vi "Excel Report - Graph Generation.vi"() -> ()   [LabVIEW 2023]
doc: "This example shows how to insert a bar graph into an Excel workbook and to set the value number format to \"percent\"."
uses:
  <vilib>/Utility/NIReport.llb/Report Type.ctl
  <vilib>/Utility/NIReport.llb/NI_report.lvclass
  <vilib>/Utility/NIReport.llb/Excel/NI_Excel.lvclass
  <vilib>/Utility/NIReport.llb/NI_ReportGenerationCore.lvlib
panel:
  in  "Has Legend?":bool
  in  "Graph Type":i32(ring)=51 items=["xlColumnClustered"=51, "xlColumnStacked"=52, "xlColumnStacked100"=53, "xl3DColumnClustered"=54, "xl3DColumnStacked"=55, "xl3DColumnStacked100"=56, "xlBarClustered"=57, "xlBarStacked"=58, "xlBarStacked100"=59, "xl3DBarClustered"=60, "xl3DBarStacked"=61, "xl3DBarStacked100"=62, "xlLineStacked"=63, "xlLineStacked100"=64, "xlLineMarkers"=65, "xlLineMarkersStacked"=66, "xlLineMarkersStacked100"=67, "xlPieOfPie"=68, "xlPieExploded"=69, "xl3DPieExploded"=70, "xlBarOfPie"=71, "xlXYScatterSmooth"=72, "xlXYScatterSmoothNoMarkers"=73, "xlXYScatterLines"=74, "xlXYScatterLinesNoMarkers"=75, "xlAreaStacked"=76, "xlAreaStacked100"=77, "xl3DAreaStacked"=78, "xl3DAreaStacked100"=79, "xlDoughnutExploded"=80, "xlRadarMarkers"=81, "xlRadarFilled"=82, "xlSurface"=83, "xlSurfaceWireframe"=84, "xlSurfaceTopView"=85, "xlSurfaceTopViewWireframe"=86, "xlBubble"=15, "xlBubble3DEffect"=87, "xlStockHLC"=88, "xlStockOHLC"=89, "xlStockVHLC"=90, "xlStockVOHLC"=91, "xlCylinderColClustered"=92, "xlCylinderColStacked"=93, "xlCylinderColStacked100"=94, "xlCylinderBarClustered"=95, "xlCylinderBarStacked"=96, "xlCylinderBarStacked100"=97, "xlCylinderCol"=98, "xlConeColClustered"=99, "xlConeColStacked"=100, "xlConeColStacked100"=101, "xlConeBarClustered"=102, "xlConeBarStacked"=103, "xlConeBarStacked100"=104, "xlConeCol"=105, "xlPyramidColClustered"=106, "xlPyramidColStacked"=107, "xlPyramidColStacked100"=108, "xlPyramidBarClustered"=109, "xlPyramidBarStacked"=110, "xlPyramidBarStacked100"=111, "xlPyramidCol"=112, "xl3DColumn"=-4100, "xlLine"=4, "xl3DLine"=-4101, "xl3DPie"=-4102, "xlPie"=5, "xlXYScatter"=-4169, "xl3DArea"=-4098, "xlArea"=1, "xlDoughnut"=-4120, "xlRadar"=-4151]
  in  "Month":string[](array[string])=["Jan", "Feb", "Mar", "Apr", "May"]
  in  "Relative Humidity":dbl[][](array[numeric])=[[0.54, 0.65, 0.56, 0.5, 0.45]]
  in  "Window State":enum16{"maximized", "minimized", "normal"}(ring)
  # "Overview: This example shows how to insert a graph into an Excel spreadsheet and to set the value number format to \"percent\".\nRequirements: Report Generation Toolkit, Microsoft Excel\nInstructions:\nRun the VI and observe the building of the Excel spreadsheet.\n\nNote: Some Graph Types do not work with this data set (Bubble, Surface, Stock)."
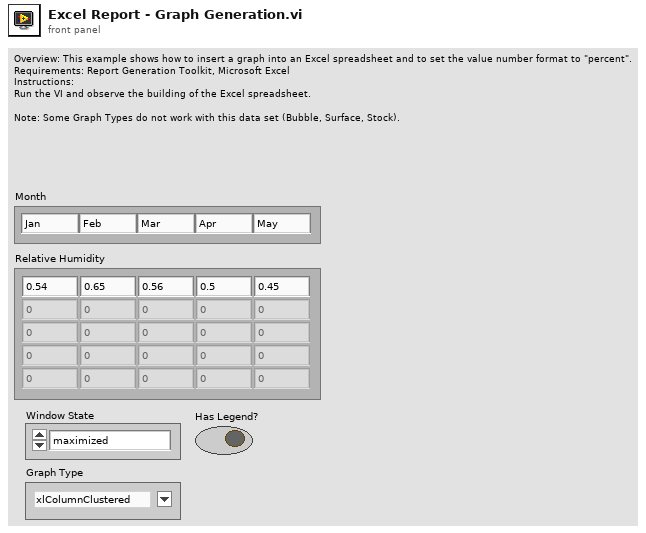
[diagram p1: front panel]
types:
  T1 = typedef "NI_ReportGenerationCore.lvlib/Report Type.ctl" = enum16{"HTML", "Word", "Excel"}
  T2 = cluster{"font style":string, "bold":bool, "italic":bool, "underline":bool, "size":sgl, "color":u32}
  T3 = cluster{"left":i32, "top":i32, "height":dbl, "width":dbl}
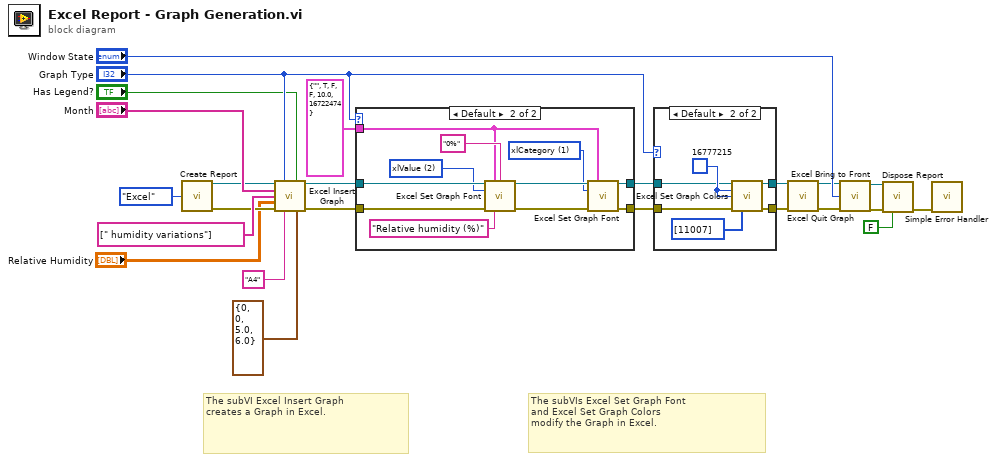
[diagram p0: block diagram]
diagram:
  # "The subVIs Excel Set Graph Font \nand Excel Set Graph Colors \nmodify the Graph in Excel."
  # "The subVI Excel Insert Graph \ncreates a Graph in Excel."
  n1 = call <vilib>:"Create Report.vi"("report type"=Report_Type."Excel" ("Report Type")) -> ("report out"=w12:refnum<class "NI_report.lvclass">, "error out"=w11:errorcluster)  [unwired: 13 in]
  n2 = call <vilib>:"Excel Insert Graph.vi"("report in"=w12, "graph type (col clustered)"="Graph Type", "has legend? (F)"="Has Legend?", "column headers"="Month", "row headers"=string[] [" humidity variations"], "data"="Relative Humidity", "error in (no error)"=w11, "name (\"\")"="A4" ("name (\"\")"), "position/size"=T3 {"left"=0, "top"=0, "height"=5.0, "width"=6.0}) -> ("report out"=w4:refnum<class "NI_report.lvclass">, "error out"=w5:errorcluster)  [unwired: 5 in]
  n3 = case shown="Default" "Graph Type" {
    tunnel: w4 -> [w26 w37]
    tunnel: w5 -> [w25 w36]
    tunnel: [w26 w34] -> w7
    tunnel: [w25 w33] -> w6
    tunnel: T2 {"font style"="", "bold"=TRUE, "italic"=FALSE, "underline"=FALSE, "size"=10.0, "color"=16722474} ("axis font") -> [_ w27]
    frame -4151, -4120, -4102, 5, 68..71, 80..82 {
      # "These Graph Types are not supported"
    }
    frame Default {
      w31 = 2 items=["xlCategory"=1, "xlSeriesAxis"=3, "xlValue"=2] ("type")
      w30 = 1 items=["xlCategory"=1, "xlSeriesAxis"=3, "xlValue"=2] ("type")
      n4 = call <vilib>:"Excel Set Graph Font.vi"("report in"=w37, "axis font"=w27, "number format (general)"="0%" ("number format (\"\")"), "axis type (xlCategory)"=w31, "error in (no error)"=w36, "title (\"\")"="Relative humidity (%)" ("title (\"\")")) -> ("report out"=w35:refnum<class "NI_report.lvclass">, "error out"=w32:errorcluster)  [unwired: 8 in]
      n5 = call <vilib>:"Excel Set Graph Font.vi"("report in"=w35, "axis font"=w27, "axis type (xlCategory)"=w30, "error in (no error)"=w32) -> ("report out"=w34:refnum<class "NI_report.lvclass">, "error out"=w33:errorcluster)  [unwired: 10 in]
    }
  }
  n6 = case shown="Default" "Graph Type" {
    tunnel: w7 -> [w39 w43]
    tunnel: w6 -> [w38 w42]
    tunnel: [w39 w41] -> w8
    tunnel: [w38 w40] -> w9
    frame 15, 87 {
    }
    frame Default {
      w44 = u32 16777215 ("plot area color")
      n7 = call <vilib>:"Excel Set Graph Colors.vi"("report in"=w43, "graph area color (w)"=w44, "plot area color (w)"=w44, "error in (no error)"=w42, "plot colors"=u32[] [11007]) -> ("report out"=w41:refnum<class "NI_report.lvclass">, "error out"=w40:errorcluster)  [unwired: 9 in]
    }
  }
  n8 = call <vilib>:"Excel Quit Graph.vi"("report in"=w8, "error in (no error)"=w9) -> ("report out"=w16:refnum<class "NI_report.lvclass">, "error out"=w17:errorcluster)  [unwired: 12 in]
  n9 = call <vilib>:"Excel Bring to Front.vi"("report in"=w16, "window state (maximized)"="Window State", "error in (no error)"=w17) -> ("report out"=w13:refnum<class "NI_report.lvclass">, "error out"=w15:errorcluster)  [unwired: 11 in]
  n10 = call-dynamic "Dispose Report.vi"("report in"=w13, "error in (no error)"=w15, "close report? (T)"=FALSE ("Close Report? (T)")) -> ("error out"=w24:errorcluster)  [unwired: 12 in]
  n11 = call <vilib>:"Simple Error Handler.vi"("error in (no error)"=w24) -> ()  [unwired: 4 in, 5 out]
